vi "CCImageToDcm.vi"() -> ()   [LabVIEW 2013, in "main.lvlib" / "ClearCanvasLibrary.lvlib"]
uses:
  ClearCanvasLibrary.lvlib
  <vilib>/picture/picture.llb/imagedata.ctl
  C:/Users/Simon/SkyDrive/LabView/2013/DM2020/DICOM/ClearCanvasNewBuild/ClearCanvas.Dicom.dll
  ClearCanvasNewBuild/ClearCanvas.Dicom.dll
panel:
  out "Dump 2":string
  out "output cluster":T1
  out "Dump":string
  out "ResultStatus":i32(ring) items=["Success", "Cancel", "Pending", "Warning", "Failure"]
  out "commandline":string
  in  "options":string="-v -i BMP"
  out "standard error":string
  out "standard output":string
  in  "executable":string="C:\\Users\\Simon\\Dropbox\\Medimatic\\ProjectVerLV2011\\DICOM\\dcmtk\\bin\\img2dcm.exe"
  in  "Excel._Worksheet":refnum<k7>
  in  "Excel._Application":refnum<k7>
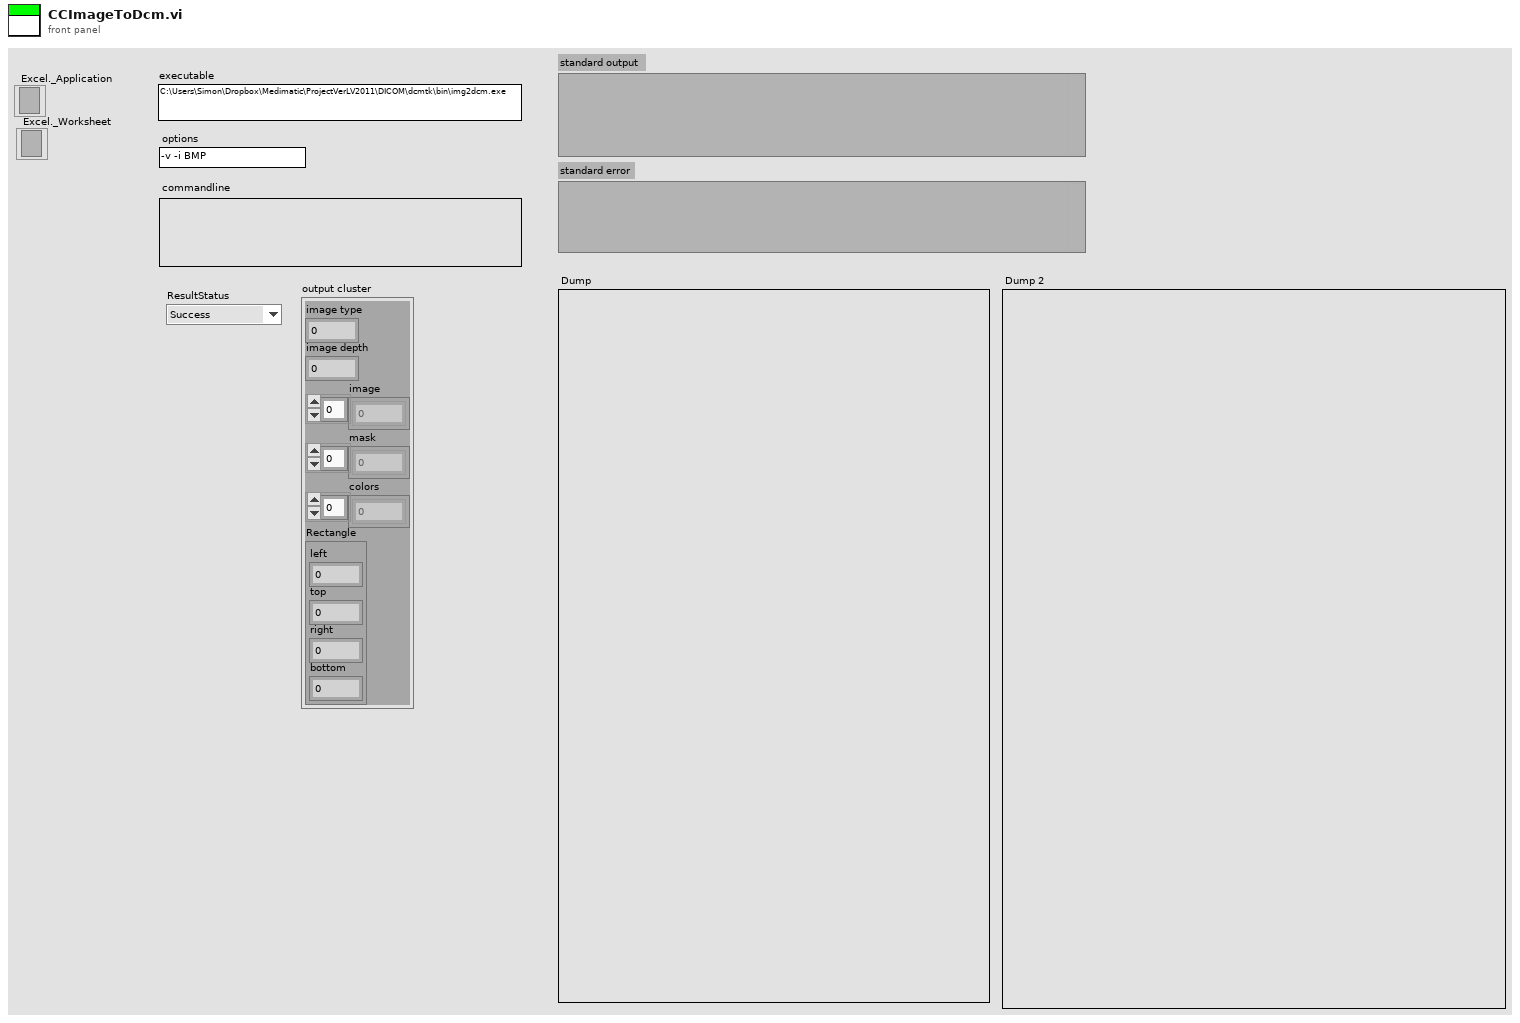
[diagram p1: front panel]
types:
  T1 = typedef "imagedata.ctl" = cluster{"image type":i32, "image depth":i32, "image":u8[], "mask":u8[], "colors":u32[], "Rectangle":cluster{"left":i16, "top":i16, "right":i16, "bottom":i16}}
  T2 = typedef "LVRectTypeDef.ctl" = cluster{"left":i16, "top":i16, "right":i16, "bottom":i16}
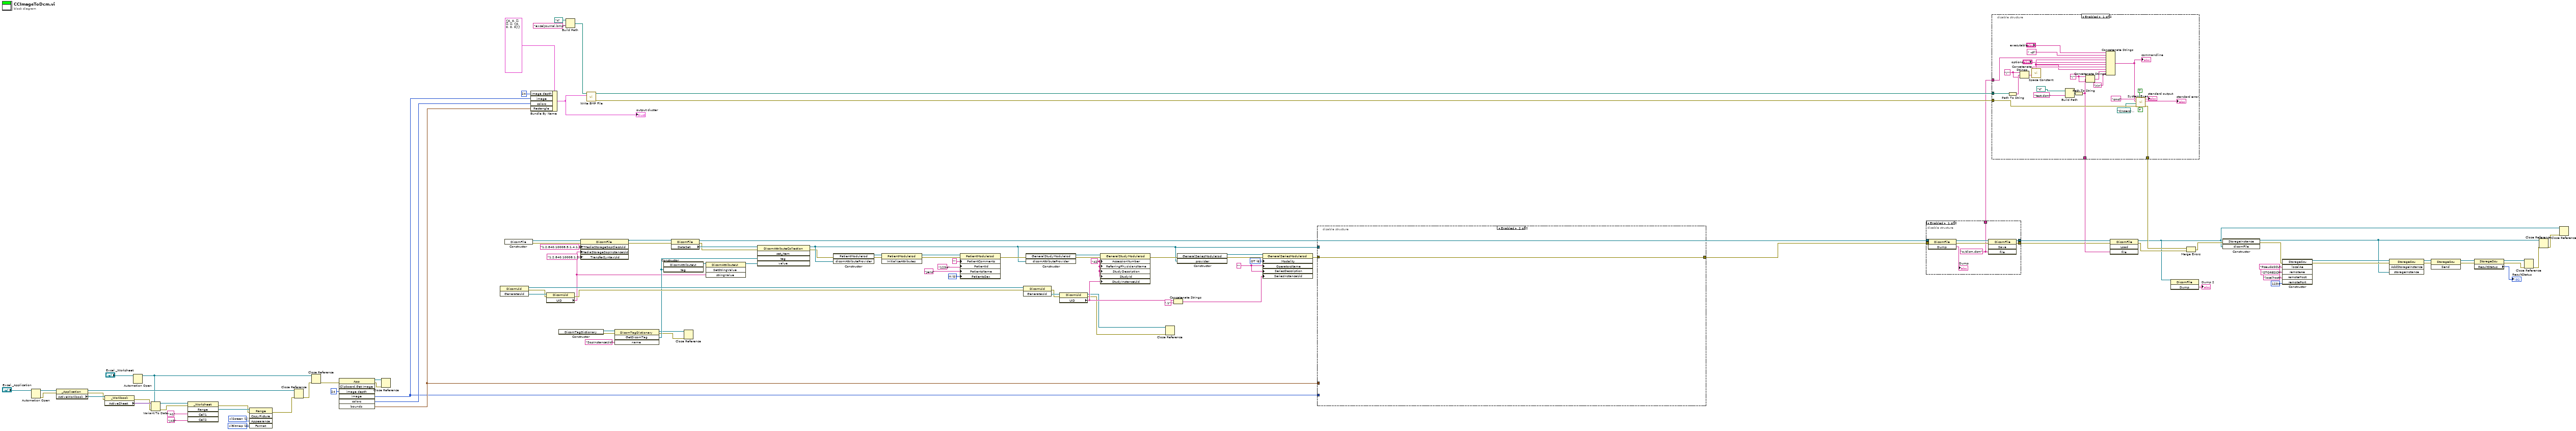
[diagram p0: block diagram]
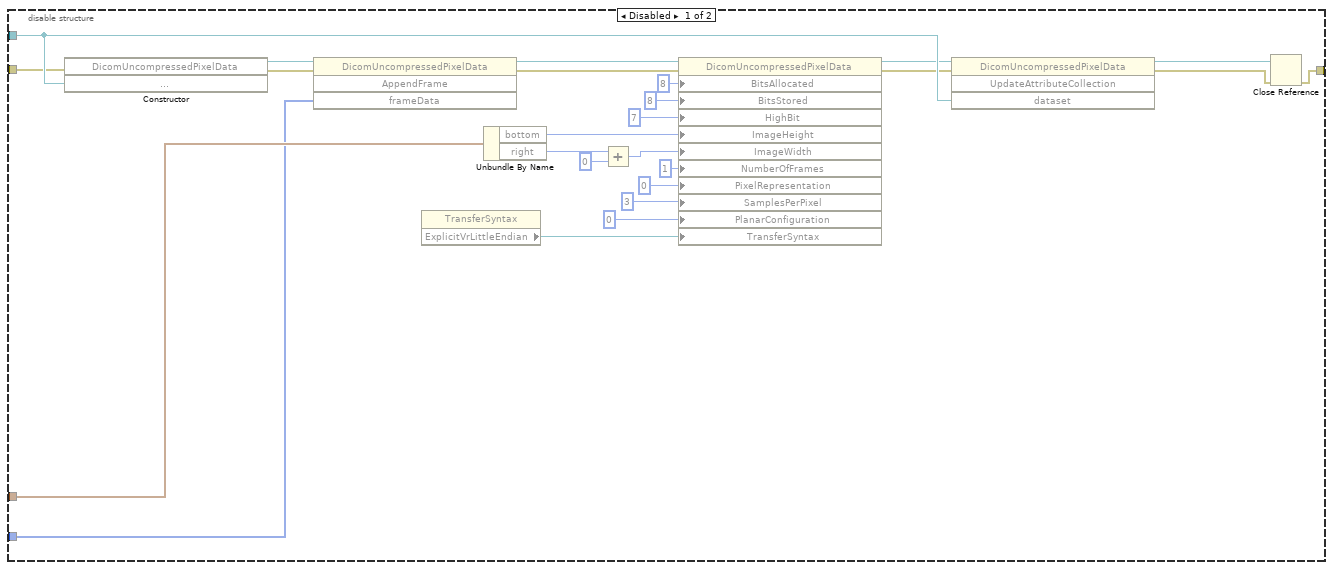
[diagram p2: hidden frame]
diagram:
  w38 = "" ("OperatorsName")
  w40 = 6 items=["None", "CR", "CT", "MR", "NM", "US", "OT", "BI", "CD", "DD", "DG", "ES", "LS", "PT", "RG", "ST", "TG", "XA", "RF", "RTImage", "RTDose", "RTStruct", "RTPlan", "RTRecord", "HC", "DX", "MG", "IO", "PX", "GM", "SM", "XC", "PR", "AU", "Ecg", "Eps", "HD", "SR", "Ivus", "OP", "Smr", "Oct", "Opr", "Opv", "Opm", "KO", "Seg", "Reg", "DS", "CF", "DF", "VF", "AS", "CS", "EC", "LP", "FA", "CP", "DM", "FS", "MA", "MS"] ("Modality")
  w43 = "42" ("AccessionNumber")
  w48 = 0 items=["M", "F", "O", "None"] ("PatientsSex")
  w106 = 2 items=["xlBitmap"=2, "xlPicture"=-4147] ("Format")
  w107 = 1 items=["xlPrinter"=2, "xlScreen"=1] ("Appearance")
  n1 = Automation Open(Automation Refnum="Excel._Application") -> (Automation Refnum=w93:refnum<k7>, error out=w92:errorcluster)  [unwired: 3 in]
  n2 = property class="_Application"(reference=w93, error in=w92) -> (reference out=w100:refnum<k7>, error out=w101:errorcluster, "ActiveWorkbook"=w110:refnum<k7>)
  n3 = property class="_Workbook"(reference=w110, error in=w101) -> (error out=w96:errorcluster, "ActiveSheet"=w103:variant)  [unwired: 1 out]
  n4 = Automation Open(Automation Refnum="Excel._Worksheet") -> (Automation Refnum=w95:refnum<k7>)  [unwired: 3 in, 1 out]
  n5 = Variant To Data(error in=w96, type=w95, Variant=w103) -> (data=w102:refnum<k7>, error out=w97:errorcluster)
  n6 = invoke class="_Worksheet" method="Range"(reference=w102, error in=w97, "Cell1"="A1", "Cell2"="J43") -> (error out=w98:errorcluster, "Range"=w108:refnum<k7>)  [unwired: 1 in, 3 out]
  n7 = invoke class="Range" method="CopyPicture"(reference=w108, error in=w98, "Appearance"=w107, "Format"=w106) -> (error out=w99:errorcluster)  [unwired: 1 in, 4 out]
  n8 = Close Reference(reference=w100, error in (no error)=w99) -> (error out=w94:errorcluster)
  n9 = Close Reference(reference=w95, error in (no error)=w94) -> (error out=w91:errorcluster)
  n10 = invoke class="App" method="Clipboard.Get Image"(error in=w91, "image depth"=24 ("Image Depth")) -> (reference out=w90:refnum<vi>, error out=w89:errorcluster, "image"=w8:u8[], "colors"=w75:u32[], "bounds"=w84:T2)  [unwired: 5 in, 2 out]
  n11 = Close Reference(reference=w90, error in (no error)=w89) -> ()  [unwired: 1 out]
  n12 = invoke class="DicomUid" method="GenerateUid"() -> (reference out=w32:refnum<k24>, error out=w82:errorcluster, "GenerateUid"=w83:refnum<k24>)  [unwired: 3 in]
  n13 = constructor class="DicomFile"() -> (reference out=w87:refnum<k24>, error out=w85:errorcluster)  [unwired: 3 in, 1 out]
  n14 = Bundle By Name(cluster=T1 {"image type"=0, "image depth"=0, "image"=[], "mask"=[], "colors"=[], "Rectangle"={"left"=0, "top"=0, "right"=0, "bottom"=0}} ("image data"), "image depth"=24, "image"=w8, "colors"=w75, "Rectangle"=w84) -> (w74:T1)
  "output cluster" <- w74
  n15 = property class="DicomUid"(reference=w83, error in=w82) -> (error out=w30:errorcluster, "UID"=w14:string)  [unwired: 1 out]
  n16 = constructor class="DicomTagDictionary"() -> (reference out=w19:refnum<k24>, error out=w11:errorcluster)  [unwired: 3 in, 1 out]
  n17 = Build Path(base path=path "c:/", name or relative path="excelJournal.bmp") -> (appended path=w80:path)
  n18 = property class="DicomFile"(reference=w87, error in=w85, "MediaStorageSopClassUid"="1.2.840.10008.5.1.4.1.1.7" ("uid"), "MediaStorageSopInstanceUid"=w14, "TransferSyntaxUid"="1.2.840.10008.1.2.1") -> (reference out=w23:refnum<k24>, error out=w22:errorcluster)
  n19 = call <vilib>:"Write BMP File.vi"("image data"=w74, "path to BMP file"=w80) -> ("error out"=w72:errorcluster, "path"=w73:path)  [unwired: 8 in]
  n20 = invoke class="DicomTagDictionary" method="GetDicomTag"(reference=w19, error in=w11, "name"="SopInstanceUid") -> (reference out=w13:refnum<k24>, error out=w12:errorcluster, "GetDicomTag"=w17:refnum<k24>)  [unwired: 1 in, 1 out]
  n21 = constructor class="DicomAttributeUI"("tag"=w17) -> (reference out=w16:refnum<k24>)  [unwired: 3 in, 3 out]
  n22 = property class="DicomFile"(reference=w23, error in=w22) -> (reference out=w76:refnum<k24>, error out=w10:errorcluster, "DataSet"=w21:refnum<k24>)
  n23 = Close Reference(reference=w13, error in (no error)=w12) -> ()  [unwired: 1 out]
  n24 = invoke class="DicomAttributeUI" method="SetStringValue"(reference=w16, "stringValue"=w14) -> (reference out=w15:refnum<k24>)  [unwired: 2 in, 3 out]
  n25 = invoke class="DicomAttributeCollection" method="set_Item"(reference=w21, error in=w10, "tag"=w17, "value"=w15) -> (reference out=w20:refnum<k24>, error out=w9:errorcluster)  [unwired: 1 in, 3 out]
  n26 = constructor class="PatientModuleIod"(error in=w9, "dicomAttributeProvider"=w20) -> (reference out=w55:refnum<k24>, error out=w54:errorcluster)  [unwired: 2 in, 2 out]
  n27 = invoke class="PatientModuleIod" method="InitializeAttributes"(reference=w55, error in=w54) -> (reference out=w53:refnum<k24>, error out=w52:errorcluster)  [unwired: 1 in, 1 out]
  n28 = property class="PatientModuleIod"(reference=w53, error in=w52, "PatientComments"="", "PatientId"="1234", "PatientsName"="Jens", "PatientsSex"=w48) -> (error out=w47:errorcluster)  [unwired: 1 out]
  n29 = invoke class="DicomUid" method="GenerateUid"(reference=w32, error in=w30) -> (error out=w29:errorcluster, "GenerateUid"=w31:refnum<k24>)  [unwired: 1 in, 1 out]
  n30 = constructor class="GeneralStudyModuleIod"(error in=w47, "dicomAttributeProvider"=w20) -> (reference out=w46:refnum<k24>, error out=w44:errorcluster)  [unwired: 2 in, 2 out]
  n31 = property class="DicomUid"(reference=w31, error in=w29) -> (reference out=w34:refnum<k24>, error out=w33:errorcluster, "UID"=w37:string)
  n32 = property class="GeneralStudyModuleIod"(reference=w46, error in=w44, "AccessionNumber"=w43, "ReferringPhysiciansName"=w43, "StudyDescription"=w43, "StudyId"=w43, "StudyInstanceUid"=w37) -> (error out=w42:errorcluster)  [unwired: 1 out]
  n33 = Close Reference(reference=w34, error in (no error)=w33) -> ()  [unwired: 1 out]
  n34 = Concatenate Strings(w37, ".1" ("string")) -> (w35:string)
  n35 = constructor class="GeneralSeriesModuleIod"(error in=w42, "provider"=w20) -> (reference out=w45:refnum<k24>, error out=w41:errorcluster)  [unwired: 2 in, 2 out]
  n36 = property class="GeneralSeriesModuleIod"(reference=w45, error in=w41, "Modality"=w40, "OperatorsName"=w38, "SeriesDescription"=w38, "SeriesInstanceUid"=w35) -> (error out=w39:errorcluster)  [unwired: 1 out]
  n37 = disable-structure shown="Enabled" {
    disable-tunnel: w84 -> [w130 _]
    disable-tunnel: [w113 w137] -> w28
    disable-tunnel: w20 -> [w124 _]
    disable-tunnel: w39 -> [w123 w137]
    disable-tunnel: w8 -> [w116 _]
    frame Disabled {
      n38 = constructor class="DicomUncompressedPixelData"(error in=w123, "collection"=w124) -> (reference out=w122:refnum<k24>, error out=w121:errorcluster)  [unwired: 2 in, 2 out]
      n39 = invoke class="DicomUncompressedPixelData" method="AppendFrame"(reference=w122, error in=w121, "frameData"=w116) -> (reference out=w120:refnum<k24>, error out=w119:errorcluster)  [unwired: 1 in, 2 out]
      n40 = property class="TransferSyntax"() -> ("ExplicitVrLittleEndian"=w112:refnum<k24>)  [unwired: 2 in, 2 out]
      n41 = Unbundle By Name(w130) -> ("bottom"=w128:i16, "right"=w127:i16)
      n42 = Add(x=w127, y=i16 0) -> (x+y=w126:i16)
      n43 = property class="DicomUncompressedPixelData"(reference=w120, error in=w119, "BitsAllocated"=u16 8, "BitsStored"=u16 8, "HighBit"=u16 7, "ImageHeight"=w128, "ImageWidth"=w126, "NumberOfFrames"=1, "PixelRepresentation"=u16 0, "SamplesPerPixel"=u16 3, "PlanarConfiguration"=u16 0, "TransferSyntax"=w112) -> (reference out=w118:refnum<k24>, error out=w117:errorcluster)
      n44 = invoke class="DicomUncompressedPixelData" method="UpdateAttributeCollection"(reference=w118, error in=w117, "dataset"=w124) -> (reference out=w115:refnum<k24>, error out=w114:errorcluster)  [unwired: 1 in, 2 out]
      n45 = Close Reference(reference=w115, error in (no error)=w114) -> (error out=w113:errorcluster)
    }
    frame Enabled {
    }
  }
  n46 = disable-structure shown="Enabled" {
    disable-tunnel: w28 -> [w145 w146]
    disable-tunnel: w76 -> [w144 w147]
    disable-tunnel: [w143 w146] -> w4
    disable-tunnel: [w142 w147] -> w7
    disable-tunnel: [w138 _] -> w27
    frame Enabled {
      w138 = "c:/dicm.dcm" ("file")
      n47 = invoke class="DicomFile" method="Dump"(reference=w144, error in=w145) -> (reference out=w141:refnum<k24>, error out=w140:errorcluster, "Dump"=→"Dump":string)  [unwired: 1 in]
      n48 = invoke class="DicomFile" method="Save"(reference=w141, error in=w140, "file"=w138) -> (reference out=w142:refnum<k24>, error out=w143:errorcluster)  [unwired: 1 in, 2 out]
    }
    frame Disabled {
    }
  }
  n49 = disable-structure shown="Enabled" {
    disable-tunnel: w72 -> [w167 w173]
    disable-tunnel: w73 -> [w166 _]
    disable-tunnel: w27 -> [w150 _]
    disable-tunnel: [w149 w173] -> w26
    disable-tunnel: [w148 _] -> w5
    frame Enabled {
      w157 = "\"" ("string")
      w164 = "\"" ("string")
      n50 = Path To String(path=w166) -> (string=w165:string)
      n51 = Concatenate Strings(w164, w165, w164) -> (w163:string)
      n52 = call <vilib>:"Space Constant.vi"() -> ("String"=w151:string)
      n53 = Build Path(base path=path "c:/", name or relative path="test.dcm") -> (appended path=w156:path)
      n54 = Path To String(path=w156) -> (string=w148:string)
      n55 = Concatenate Strings(w157, w148, w157) -> (w154:string)
      n56 = Concatenate Strings("executable", " -df ", w150, w151, "options", w151, w163, w151, w154, "\r\n") -> (w161:string)
      "commandline" <- w161
      n57 = call <vilib>:"System Exec.vi"("run minimized? (F)"=TRUE, "wait until completion? (T)"=TRUE, "error in (no error)"=w167, "working directory"=path "C:/Users/Simon/Dropbox/Medimatic/ProjectVerLV2011/DICOM/dcmtk/bin", "standard input"=w161, "command line"="cmd") -> ("error out"=w149:errorcluster, "standard error"=→"standard error":string, "standard output"=→"standard output":string)  [unwired: 2 in, 1 out]
    }
    frame Disabled {
    }
  }
  n58 = invoke class="DicomFile" method="Load"(reference=w7, error in=w4, "file"=w5) -> (reference out=w2:refnum<k24>, error out=w3:errorcluster)  [unwired: 1 in, 2 out]
  n59 = invoke class="DicomFile" method="Dump"(reference=w2) -> ("Dump"=→"Dump 2":string)  [unwired: 2 in, 2 out]
  n60 = Merge Errors(w26, w3) -> (w25:errorcluster)
  n61 = constructor class="StorageInstance"(error in=w25, "dicomFile"=w2) -> (reference out=w6:refnum<k24>, error out=w64:errorcluster)  [unwired: 2 in, 2 out]
  n62 = constructor class="StorageScu"(error in=w64, "localAe"="PseudoSCU", "remoteAe"="STORESCP", "remoteHost"="localhost", "remotePort"=1234) -> (reference out=w71:refnum<k24>, error out=w65:errorcluster)  [unwired: 2 in, 5 out]
  n63 = invoke class="StorageScu" method="AddStorageInstance"(reference=w71, error in=w65, "storageInstance"=w6) -> (reference out=w59:refnum<k24>, error out=w58:errorcluster)  [unwired: 1 in, 2 out]
  n64 = invoke class="StorageScu" method="Send"(reference=w59, error in=w58) -> (reference out=w57:refnum<k24>, error out=w56:errorcluster)  [unwired: 1 in, 1 out]
  n65 = property class="StorageScu"(reference=w57, error in=w56) -> (reference out=w61:refnum<k24>, error out=w62:errorcluster, "ResultStatus"=→"ResultStatus":i32)
  n66 = Close Reference(reference=w61, error in (no error)=w62) -> (error out=w66:errorcluster)
  n67 = Close Reference(reference=w6, error in (no error)=w66) -> (error out=w63:errorcluster)
  n68 = Close Reference(reference=w2, error in (no error)=w63) -> ()  [unwired: 1 out]
